vi "LF2R IDE Launcher.vi"   [LabVIEW 2018]
uses:
  Source/Actor/Main Panel/LF2R IDE/Main Panel.lvclass
  C:/Program Files (x86)/National Instruments/LabVIEW 2018/vi.lib/MGI/Panel Manager/Panel Actor/Panel Actor/Panel Actor.lvclass
  <vilib>/MGI/Panel Manager/Panel/Window Position/Reference Position/Ref Top Level/Ref Top Level.lvclass
  C:/Program Files (x86)/National Instruments/LabVIEW 2018/vi.lib/MGI/Panel Manager/Panel/Window Position/Window Position.lvclass
  <vilib>/MGI/Panel Manager/Panel/Window Position/Reference Position/Ref Top Level/Ref Top Level.vi
  <vilib>/MGI/Panel Manager/Panel Actor/Panel Actor/Launch Root Panel Window.vi
  <vilib>/MGI/Panel Manager/Panel Actor/Panel Actor/Panel Actor.lvclass
  <vilib>/MGI/Panel Manager/Panel/Panel.lvlib
  C:/Program Files (x86)/National Instruments/LabVIEW 2018/vi.lib/MGI/Panel Manager/Panel/Window Position/Reference Position/Reference Position.lvclass
  D:/project/hobby/LabVIEW/LF2R/LabVIEW/Source/Actor/Framework/Framework/Framework.lvclass
  C:/Program Files (x86)/National Instruments/LabVIEW 2018/vi.lib/MGI/Monitored Actor/Monitored Actor/Monitored Actor/Monitored Actor.lvclass
  C:/Program Files (x86)/National Instruments/LabVIEW 2018/vi.lib/ActorFramework/Actor/Actor.lvclass
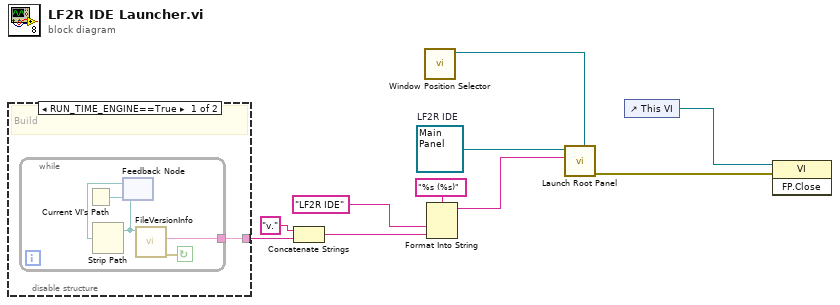
[diagram p0: block diagram]
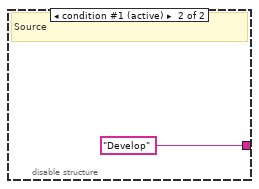
[diagram p2: hidden frame]
diagram:
  w10 = refnum<class "Main Panel.lvclass"> refnum  # LF2R IDE
  n1 = disable-structure shown="RUN_TIME_ENGINE==True" {
    disable-tunnel: [w11 "Develop" ("File Version Info")] -> w8
    frame condition #0 {
      # "Build"
      n2 = while {
        tunnel: [w12] -> w11
        stop <- w13 continue-if-true
        n3 = Current VI's Path() -> (path=w16:path)
        n4 = feedback #1(w16) -> (w15:path)
        n5 = Strip Path(path=w15) -> (stripped path=w14:path)  [unwired: 1 out]
        n6 = feedback-in #1(w14) -> ()
        n7 = call <vilib>:"FileVersionInfo.vi"("Application Path in"=w14) -> ("error out"=w13:errorcluster, "File Version Info"=w12:string)  [unwired: 7 in, 2 out]
      }
    }
    frame condition #1 (active) {
      # "Source"
    }
  }
  n8 = Concatenate Strings("v." ("string"), w8) -> (w4:string)
  n9 = call-poly <vilib>:"Window Position Selector.vi"() -> ("Ref Top Level out"=w9:refnum<class "Ref Top Level.lvclass">)  [unwired: 10 in, 1 out]
  n10 = Format Into String(format string="%s (%s)", "LF2R IDE" ("Start up Title"), w4) -> (resulting string=w3:string)  [unwired: 2 in, 1 out]
  n11 = call-poly <vilib>:"Launch Root Panel.vi"("Window Position (Maximize First Call)"=w9, "Title"=w3, "Panel Actor in"=w10) -> ("Error Out"=w1:errorcluster)  [unwired: 7 in, 1 out]
  n12 = control-ref of="This VI"() -> (w2:refnum<vi>)
  n13 = invoke class="VI" method="FP.Close"(reference=w2, error in=w1) -> ()  [unwired: 1 in, 3 out]
